vi "GetVideoDriver.vi"(8 "No Error":errorcluster, 11 "Index":i32) -> (0 "Error Out":errorcluster, 3 "Video Driver":string)   [LabVIEW 2024, in "SDL3.lvlib" / "Video.lvlib"]
doc: "<B>Summary</B>\nGet the name of a built in video driver.\n\n<B>Remarks</B>\nThe video drivers are presented in the order in which they are normally checked during initialization.\n\nThe names of drivers are all simple, low-ASCII identifiers, like \"cocoa\", \"x11\" or \"windows\". These never have Unicode characters, and are not meant to be proper names."
uses:
  Video.lvlib
  Lib/SDL3-32.dll
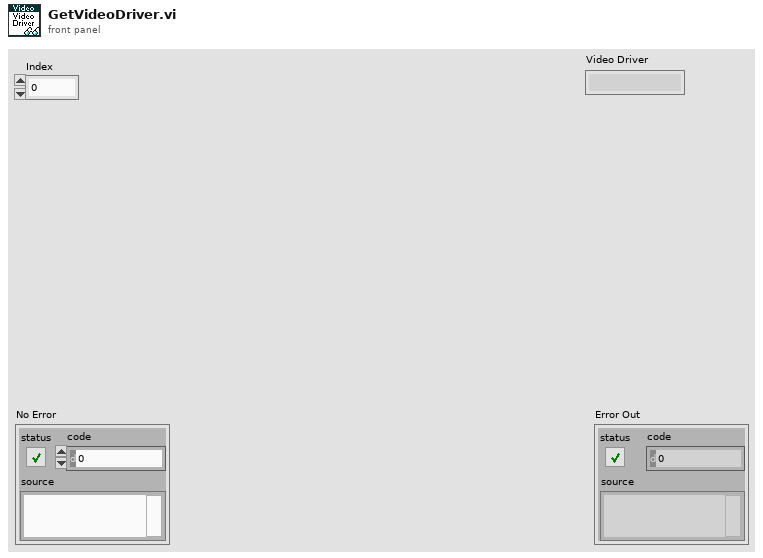
[diagram p1: front panel]
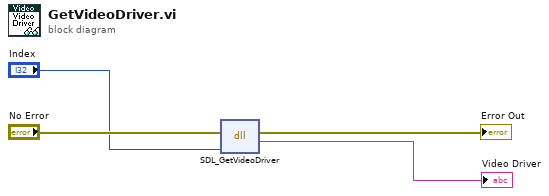
[diagram p0: block diagram]
diagram:
  n1 = dll-call lib="C:/Users/Thomas/Documents/Projects/LV-SDL3/Lib/SDL3-*.*" fn="SDL_GetVideoDriver"(error in="No Error", "index"="Index") -> (error out=→"Error Out":errorcluster, "return type"=→"Video Driver":string)  [unwired: 3 in, 1 out]
